vi "Evaluate Channel as Bit.vi"(10 "channel descriptor":T1 {"buffer offset" format="%d bytes"}, 11 "buffer in":string) -> (2 "bit":bool, 3 "buffer out":string)   [LabVIEW 2017, in "DSF Core.lvlib" / "Buffer Converter.lvclass"]
uses:
  Buffer Converter.lvclass
  Channel Descriptor.ctl
  DSF Configuration API/Public/Controls/DSF Data Type.ctl
  DSF Core.lvlib
  Buffer/Buffer.lvclass
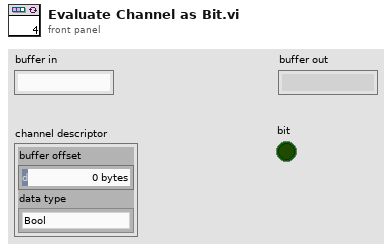
[diagram p1: front panel]
types:
  T1 = typedef "DSF Core.lvlib/Buffer.lvclass/Channel Descriptor.ctl" = cluster{"buffer offset":u64, "data type":T2}
  T2 = typedef "DSF Core.lvlib/DSF Data Type.ctl" = enum8{"Bool", "SGL", "DBL", "I8", "I16", "I32", "I64", "U8", "U16", "U32", "U64"}
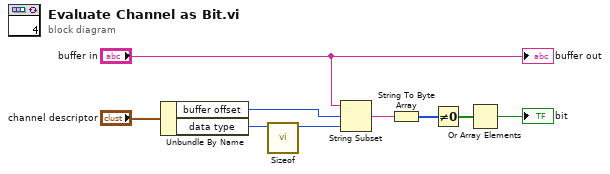
[diagram p0: block diagram]
diagram:
  n1 = Unbundle By Name("channel descriptor") -> ("buffer offset"=w9:u64, "data type"=w8:T2)
  n2 = call "Sizeof.vi"("data type"=w8) -> ("size in bytes"=w7:u64)  [unwired: 9 in, 1 out]
  n3 = String Subset(string="buffer in", offset (0)=w9, length (rest)=w7) -> (substring=w4:string)
  n4 = String To Byte Array(string=w4) -> (unsigned byte array=w6:u8[])
  n5 = Not Equal To 0?(x=w6) -> (x != 0?=w5:bool[])
  n6 = Or Array Elements(Boolean array=w5) -> (logical OR=→"bit":bool)
  "buffer out" <- "buffer in"
